vi "FisherPaykel Motor Setup 2.vi"(7 "Debug":bool, 8 "Error In":errorcluster, 9 "Motor Number":u16=130 max=255 step=1, 10 "Main Command":T1=">SMN", 11 "VISA Refnum in":refnum<visa-resource-name>) -> (0 "Error Out":errorcluster, 3 "VISA Refnum out":refnum<visa-resource-name>)   [LabVIEW 2016]
uses:
  Type Definitions/Fisher Paykel Main Command.ctl
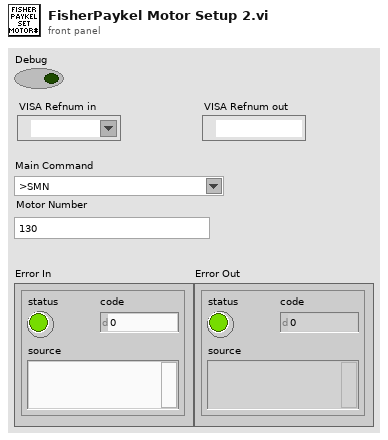
[diagram p1: front panel]
types:
  T1 = typedef "Fisher Paykel Main Command.ctl" = string
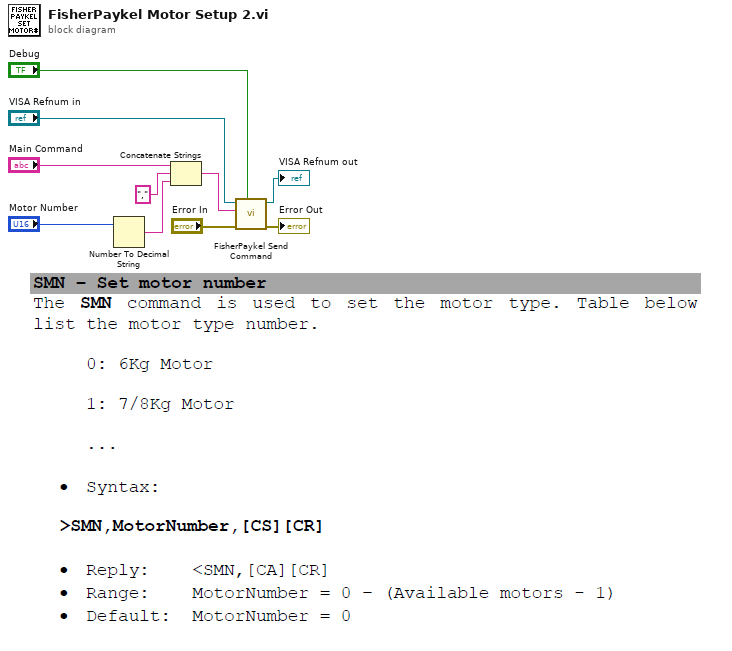
[diagram p0: block diagram]
diagram:
  n1 = Number To Decimal String(number="Motor Number") -> (decimal integer string=w7:string)  [unwired: 1 in]
  n2 = Concatenate Strings("Main Command", "," ("string"), w7) -> (w6:string)
  n3 = call "FisherPaykel Send Command.vi"("Debug"="Debug", "error in (no error)"="Error In", "Send Command"=w6, "VISA Refnum in"="VISA Refnum in") -> ("error out"=→"Error Out":errorcluster, "VISA Refnum out"=→"VISA Refnum out":refnum<visa-resource-name>)  [unwired: 5 in, 1 out]
